vi "depth to intensity.vi"(0 "Display State In":T1={"control refs"={"z offset"=refnum, "laser intensity"=refnum, "XY graph"=refnum}, "error"={"status"=FALSE, "code"=0, "source"=""}, "free-run?"=TRUE, "settings"={"fix points"=[], "A"=0.0, "lambda"=0.0, "C"=0.0}, "range (um)"=400, "interpolate?"=FALSE}, 5 "depth":dbl[unit], 9 "Container State":T4, 11 "error in (no error)":errorcluster) -> (4 "Display State Out":T1={"control refs"={"z offset"=refnum, "laser intensity"=refnum, "XY graph"=refnum}, "error"={"status"=FALSE, "code"=0, "source"=""}, "free-run?"=TRUE, "settings"={"fix points"=[], "A"=0.0, "lambda"=0.0, "C"=0.0}, "range (um)"=400, "interpolate?"=FALSE}, 6 "intensity":dbl, 15 "error out":errorcluster)   [LabVIEW 2010, in "XIntensityCompensation.xctl"]
uses:
  XIntensityCompensation.xctl
  <vilib>/_xctls/Container State.ctl
  state.ctl
  control_refs.ctl
  settings_cluster.ctl
  <vilib>/_xctls/XControlSupport.lvlib
panel:
  # "Add Controls & Indicators that form the parameters of the method here. Hook them to the connector pane. Do not delete the controls & indicators that are already hooked to the connector pane.\n \nTo setup the parameters  for this method, right click on this item in the Project Tree & select \"Configure Method...\"."
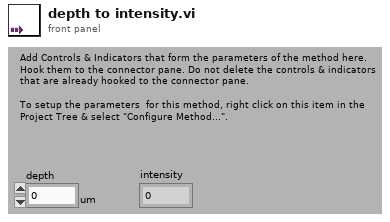
[diagram p1: front panel]
types:
  T1 = typedef "XIntensityCompensation.xctl/state.ctl" = cluster{"control refs":T2, "error":errorcluster, "free-run?":bool, "settings":T3, "range (um)":i32, "interpolate?":bool}
  T2 = typedef "XIntensityCompensation.xctl/control_refs.ctl" = cluster{"z offset":refnum<vi>, "laser intensity":refnum<vi>, "XY graph":refnum<vi>}
  T3 = typedef "XIntensityCompensation.xctl/settings_cluster.ctl" = cluster{"fix points":cluster{"depth":dbl[unit], "intensity":dbl}[], "A":dbl, "lambda":dbl[unit], "C":dbl}
  T4 = typedef "XControlSupport.lvlib/Container State.ctl" = cluster{"Indicator?":bool, "Run Mode?":bool, " Refnum":refnum<vi>}
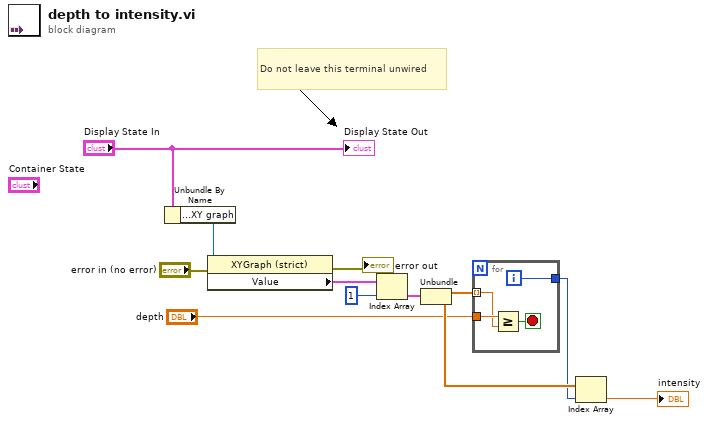
[diagram p0: block diagram]
diagram:
  # "Do not leave this terminal unwired"
  n1 = Unbundle By Name("Display State In") -> ("control refs.XY graph"=w12:refnum<vi>)
  n2 = property class="XYGraph (strict)"(reference=w12, error in="error in (no error)") -> (error out=→"error out":errorcluster, "Value"=w11:cluster{dbl[unit][], dbl[]}[])  [unwired: 1 out]
  n3 = Index Array(array=w11, index=1) -> (element=w9:cluster{dbl[unit][], dbl[]})
  n4 = Unbundle(w9) -> (w8:dbl[unit][], w7:dbl[])
  n5 = for {
    tunnel: "depth" -> [w16]
    tunnel: w8 -> [w15] mode=indexing
    tunnel: [w13] -> w5
    i -> [w13]
    stop <- w14 stop-if-true
    n6 = Greater Or Equal?(x=w16, y=w15) -> (x >= y?=w14:bool)
  }
  n7 = Index Array(array=w7, index=w5) -> (element=→"intensity":dbl)
  "Display State Out" <- "Display State In"
